vi "is Leap Year.vi"(5 "year":u16) -> (2 "lear year?":bool)   [LabVIEW 2020]
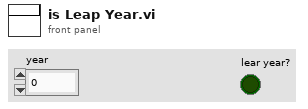
[diagram p1: front panel]
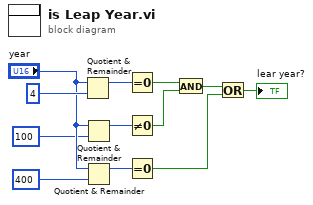
[diagram p0: block diagram]
diagram:
  n1 = Quotient & Remainder(x="year", y=u16 4) -> (x-y*floor(x/y)=w8:u16)  [unwired: 1 out]
  n2 = Quotient & Remainder(x="year", y=u16 100) -> (x-y*floor(x/y)=w6:u16)  [unwired: 1 out]
  n3 = Quotient & Remainder(x="year", y=u16 400) -> (x-y*floor(x/y)=w7:u16)  [unwired: 1 out]
  n4 = Equal To 0?(x=w8) -> (x = 0?=w5:bool)
  n5 = Not Equal To 0?(x=w6) -> (x != 0?=w4:bool)
  n6 = Equal To 0?(x=w7) -> (x = 0?=w2:bool)
  n7 = And(x=w5, y=w4) -> (x .and. y?=w3:bool)
  n8 = Or(x=w3, y=w2) -> (x .or. y?=→"lear year?":bool)
